vi "J1939 Workspace Tool.vi"() -> ()   [LabVIEW 2015, in "J1939 Workspace Object.lvlib"]
uses:
  J1939 Workspace Object.lvlib
  NationalInstruments.VeriStand.SystemStorage
  Shared/Types/Private Data.ctl
  Shared/Types/Error Cluster.ctl
  Shared/Types/Error Types.ctl
  Shared/J1939 Utilities/SubVIs/Convert CAN Arb ID to J1939 ID.vi
  <vilib>/NI Veristand/Execution/Workspace/NI_VS Workspace ExecutionAPI.lvlib
  Shared/J1939 Addon Shared.lvlib
  Shared/J1939 Utilities/J1939 Utilities.lvlib
  <vilib>/NI/VeriStand Addon Network Comm/Shared/NI VeriStand Addon Network Comm Shared.lvlib
panel:
  out "Device":string
  in  "Cluster":T1={"PGN"=65226, "DA"=0, "CD Path"="", "CD IP"=""}
  in  "Errors":bool
  in  "Tab Control":enum32{"DTCs", "Custom RQST", "RAW FRAME"}(tab)
  in  "Refresh Continuous":bool
  in  "Clear DTC":bool
  in  "Refresh DTCs":bool
  in  "DTCs":i32(listbox)
  in  "Addresses":string(tree)
  in  "Refresh Addresses":bool
  out "Response":string
  in  "Request":bool
  in  "PGN":u32
  in  "DA":u8(ring)
  in  "Clear Array":bool
  out "Priority":u8 format="%02x"
  out "SA":u8 format="%02x"
  out "PGN":u32 format="%06x"
  in  "Identifier":u32 format="%08x"
  in  "RAW":bool
  in  "Data":u8[](array[numeric])=[0, 0, 0, 0, 0, 0, 0, 0]
  in  "NIVS.System Definition Root":refnum<k24>
  in  "NIVS.Workspace Event":refnum<event-registration>
  in  "NIVS.Gateway IP Address":string
  # "Use this example as a template to create custom tools for the NI VeriStand Workspace. This example shows the use of the NI VeriStand API and UI controls to set and get data.\n\nRun this example by adding this VI as a Workspace Tool item. For Help adding Workspace Tool items, please reference the NI VeriStand Help."
  # "This is the file path to the VeriStand system definition file. You can read or write to the file using the System Definition API."
  # "This is the root reference to the active System Definition file. You could use this to read the configuration or populate a tree with channels. You are free to close this reference, but it will be closed for you if you don't."
  # "The SystemStorageUI .NET assembly provides controls to display data configured in the System Definition file."
  # "This is the IP Address of the VeriStand Gateway to which the Workspace is connected. Use this to open all the .NET Manager references. Usually the Gateway is running on localhost, but it could be running on a neighbor's machine."
  # "This registered string User Event is used to help instruct your tool to shut down when the Workspace is closing."
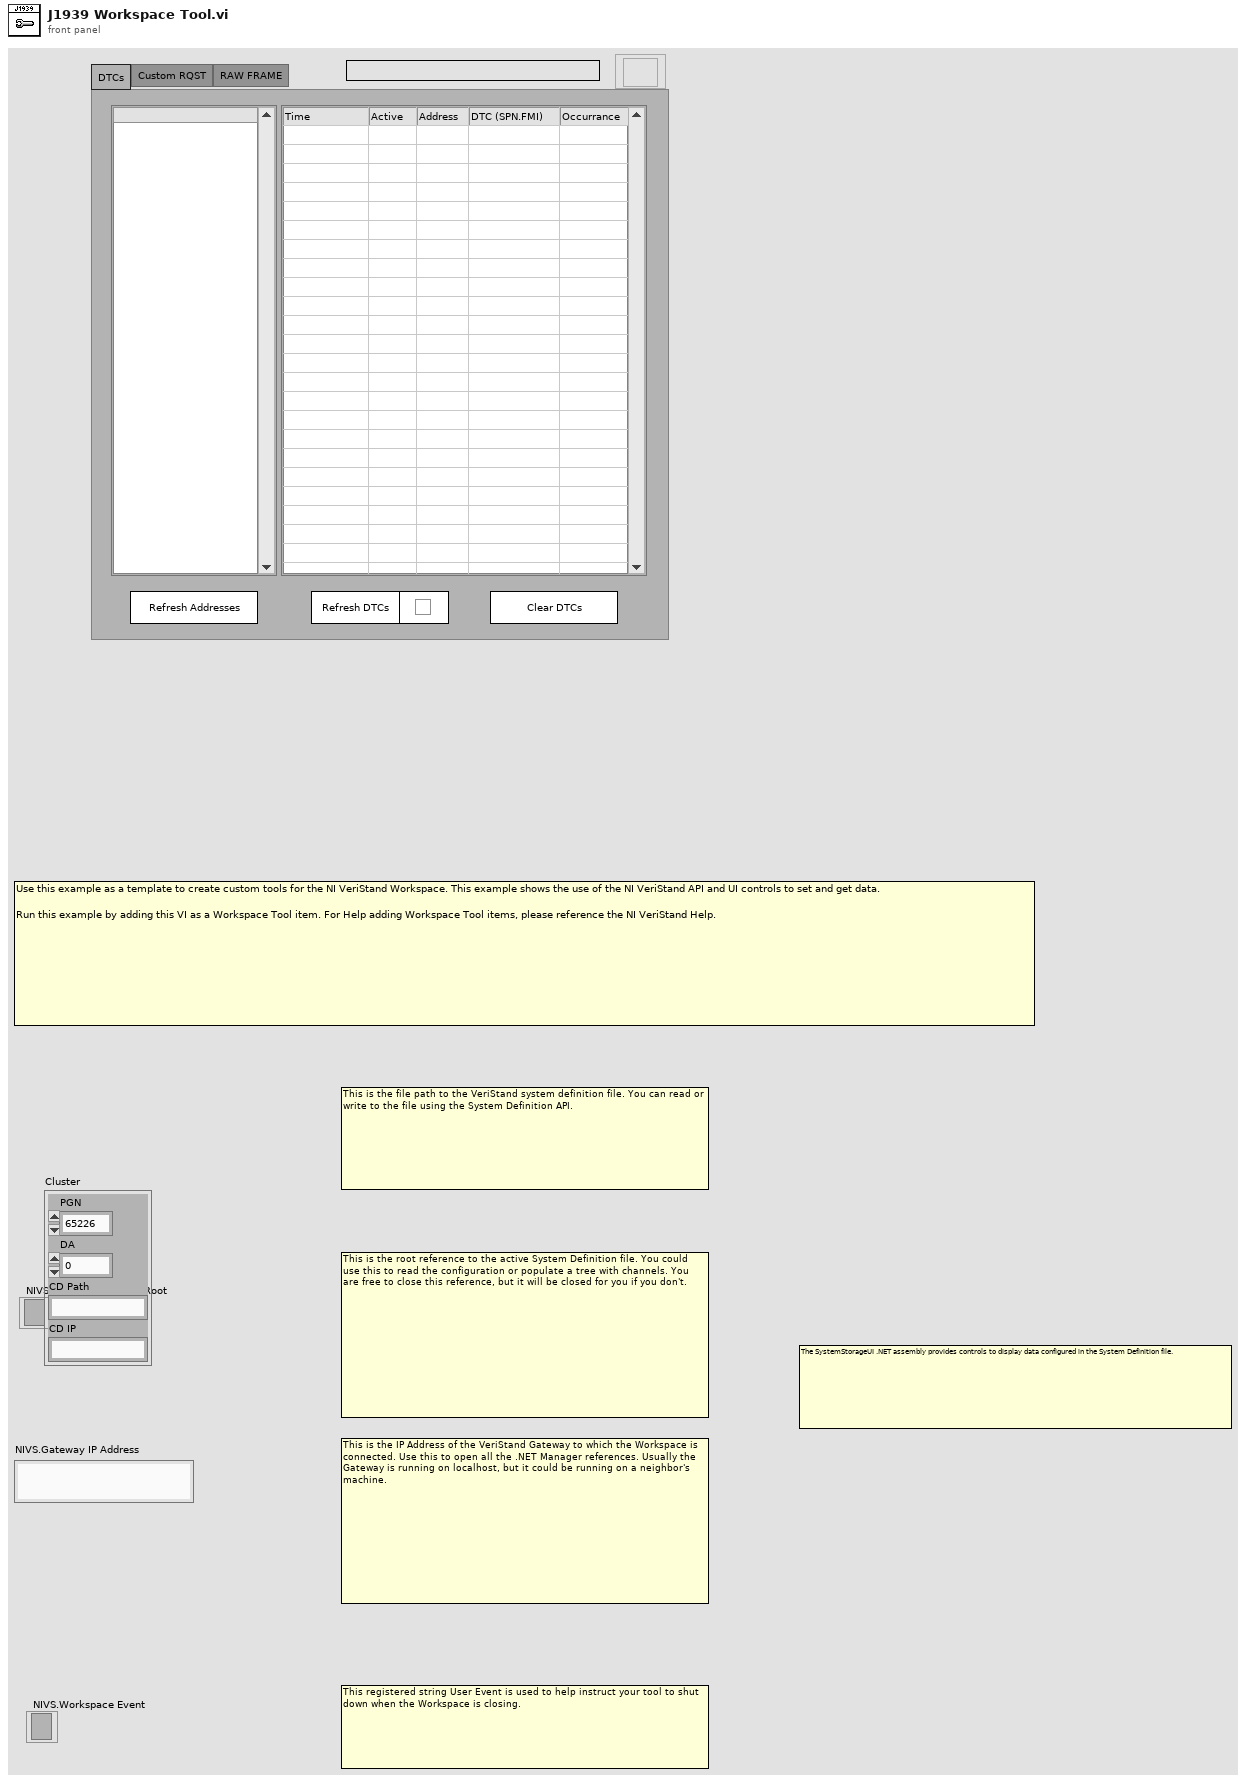
[diagram p1: front panel]
types:
  T1 = typedef "J1939 Addon Shared.lvlib/Private Data.ctl" = cluster{"PGN":u32, "DA":u8, "CD Path":string, "CD IP":string}
  T2 = typedef "J1939 Addon Shared.lvlib/Error Cluster.ctl" = cluster{"error out":errorcluster, "Enum":T3, "Address":u8, "Timestamp":timestamp}
  T3 = typedef "J1939 Addon Shared.lvlib/Error Types.ctl" = enum16{"Request", "RAW Generation", "Clear Active DTCs", "Clear Previous DTCs", "Addresses", "TLAs", "Get Active DTCs", "Get Previous DTCs"}
  T4 = typedef "NI STM.lvlib/TCP Connection Info.ctl" = cluster{"connection ID":refnum<k5>, "meta data":T5[]}
  T5 = typedef "NI STM.lvlib/MetaDataElement.ctl" = string
  T6 = typedef "NI_VS Workspace ExecutionAPI.lvlib/WorkspaceAPI.ctl" = refnum<k24>
  T7 = typedef "NI_VS Workspace ExecutionAPI.lvlib/SystemStateEventRef.ctl" = cluster{"CustDatRef":refnum<user-event>, "EvtRef":refnum<k27>, "Target State User Event":refnum<user-event>}
  T8 = typedef "NI_VS Workspace ExecutionAPI.lvlib/SystemStateRegEventRef.ctl" = refnum<event-registration>
  T9 = cluster{"NIVS.Workspace Event":refnum<event-registration>, "SystemChangeEventRef":T8}
  T10 = enum8{"Enabled", "Disabled", "Disabled and Grayed Out"}
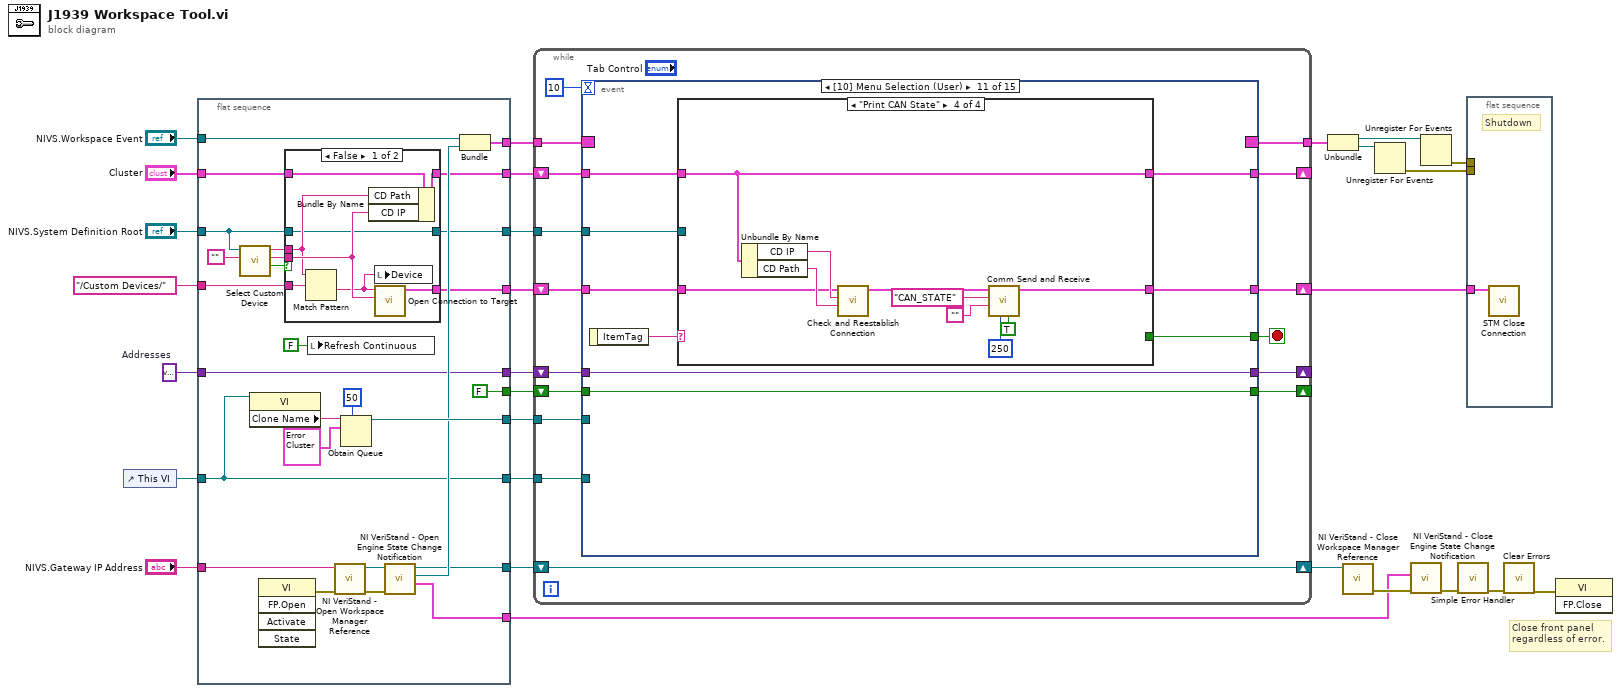
[diagram p0: block diagram]
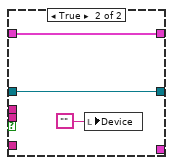
[diagram p2: hidden frame]
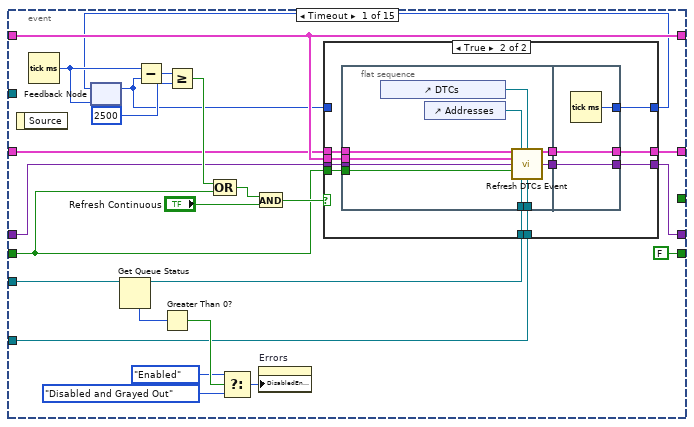
[diagram p3: hidden frame]
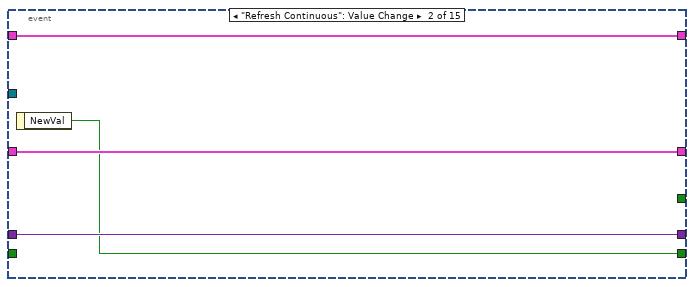
[diagram p5: hidden frame]
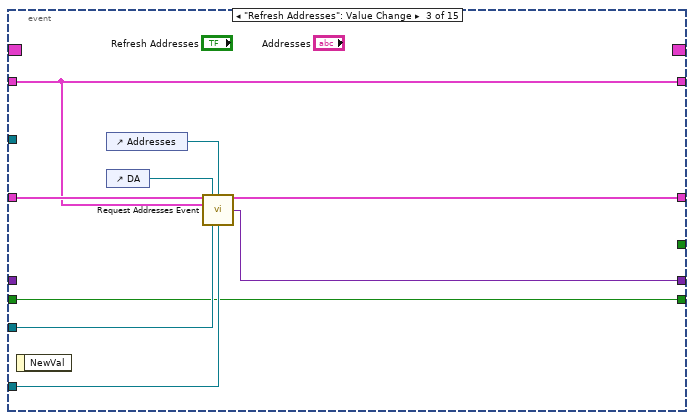
[diagram p6: hidden frame]
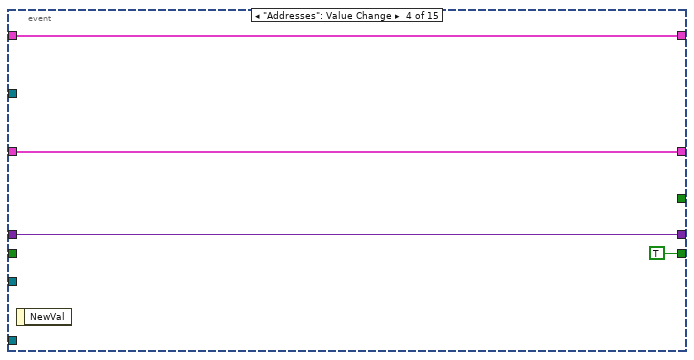
[diagram p7: hidden frame]
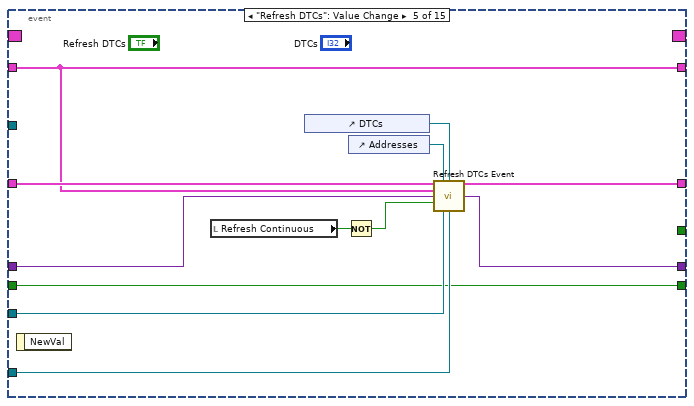
[diagram p8: hidden frame]
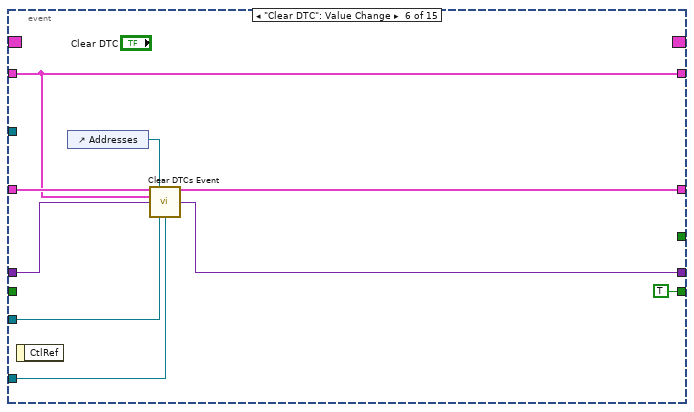
[diagram p9: hidden frame]
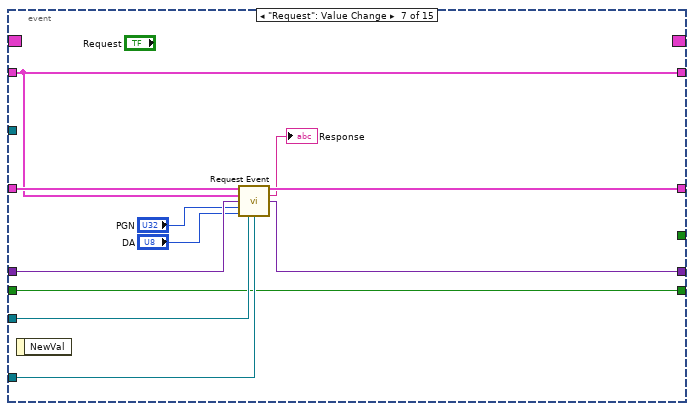
[diagram p10: hidden frame]
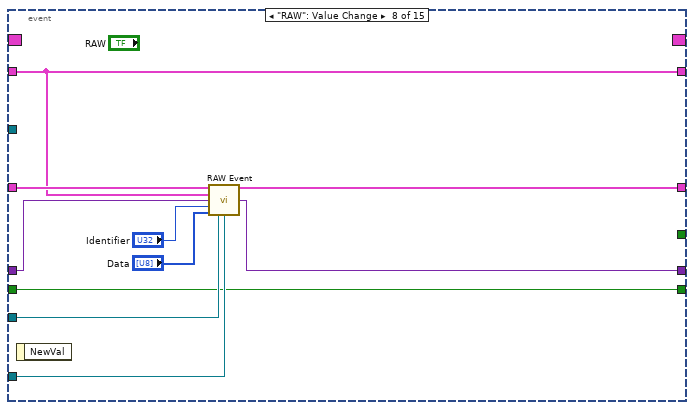
[diagram p11: hidden frame]
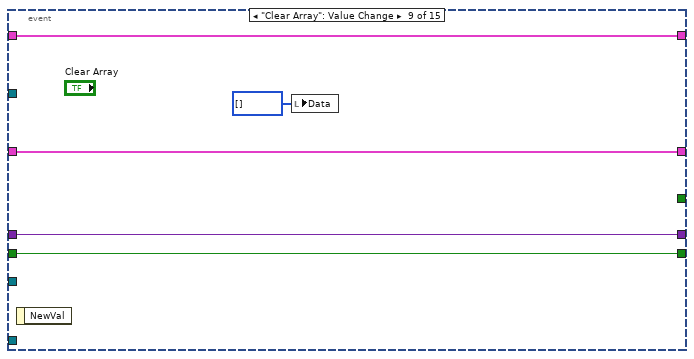
[diagram p12: hidden frame]
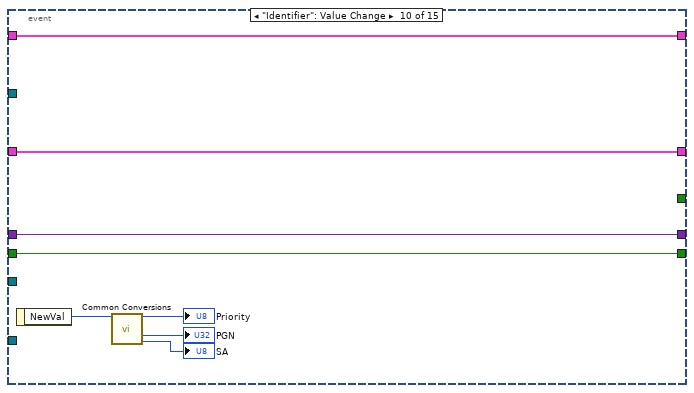
[diagram p13: hidden frame]
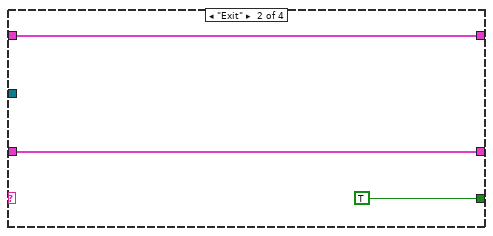
[diagram p15: hidden frame]
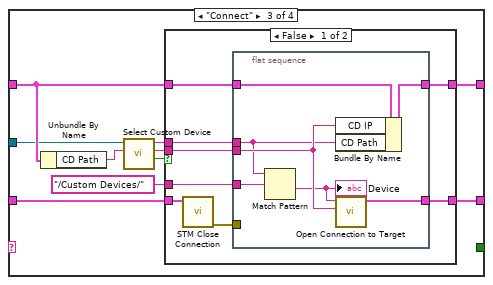
[diagram p16: hidden frame]
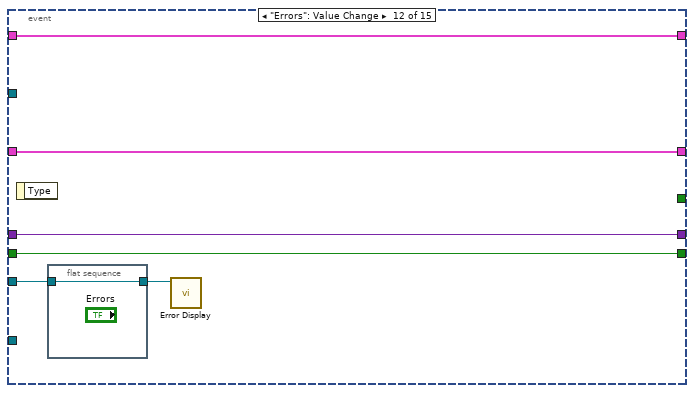
[diagram p18: hidden frame]
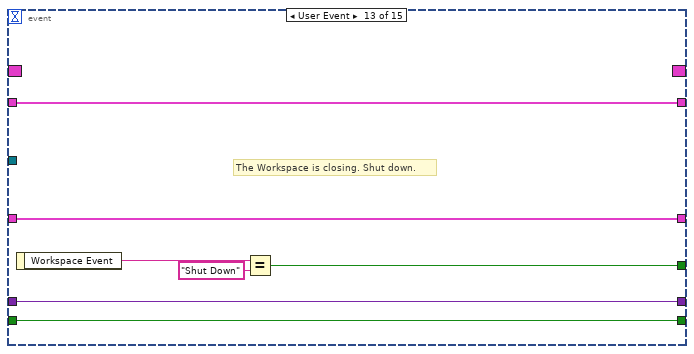
[diagram p19: hidden frame]
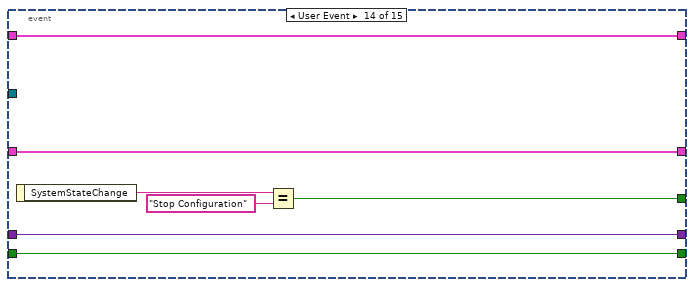
[diagram p20: hidden frame]
diagram:
  w6 = variant  # Addresses
  # "Close front panel\nregardless of error."
  n1 = control-ref of="This VI"() -> (w8:refnum<vi>)
  n2 = flat-sequence {
    tunnel: [w37] -> w28
    tunnel: [w41] -> w26
    tunnel: "NIVS.System Definition Root" -> [w31]
    tunnel: [w54] -> w25
    tunnel: [w42] -> w24
    tunnel: "NIVS.Gateway IP Address" -> [w48]
    tunnel: "NIVS.Workspace Event" -> [w46]
    tunnel: [w45] -> w20
    tunnel: [w44] -> w12
    tunnel: [w43] -> w11
    tunnel: [w39] -> w9
    tunnel: w8 -> [w42]
    tunnel: "Cluster" -> [w38]
    tunnel: w6 -> [w41]
    tunnel: [w30] -> w3
    tunnel: "/Custom Devices/" ("regular expression") -> [w35]
    tunnel: [FALSE] -> w1
    frame #0 {
      n3 = call "Select Custom Device.vi"("CD Path"="", "NIVS.System Definition Root"=w31) -> ("Cancelled?"=w32:bool, "IP Address"=w40:string, "Custom Device Path Out"=w34:string)  [unwired: 7 in]
      n4 = property class="VI"(reference=w42) -> ("Clone Name"=w55:string)  [unwired: 1 in, 2 out]
      n5 = invoke class="VI" method="FP.Open"() -> (error out=w51:errorcluster)  [unwired: 5 in, 4 out]
      n6 = case shown="False" w32 {
        tunnel: w40 -> [w63 _]
        tunnel: [w62 _] -> w39
        tunnel: w38 -> [w60 w66]
        tunnel: [w59 w66] -> w37
        tunnel: w35 -> [w58 _]
        tunnel: w34 -> [w57 _]
        tunnel: w31 -> [w56 w64]
        tunnel: [w56 w64] -> w30
        frame False {
          n7 = Match Pattern(string=w57, regular expression=w58) -> (after substring=w61:string)  [unwired: 1 in, 3 out]
          n8 = Bundle By Name(cluster=w60, "CD Path"=w57, "CD IP"=w63) -> (w59:T1)
          n9 = local write "Device"(w61) -> ()
          n10 = call "Open Connection to Target.vi"("IP Address"=w63, "TCP Service"=w61) -> ("connection info"=w62:T4)  [unwired: 8 in, 1 out]
        }
        frame True {
          n11 = local write "Device"("") -> ()
        }
      }
      n12 = local write "Refresh Continuous"(FALSE ("Refresh Continuous")) -> ()
      n13 = call <vilib>:"NI VeriStand - Open Workspace Manager Reference.vi"("error in (no error)"=w51, "Gateway IP Address (\"\": localhost)"=w48) -> ("error out"=w50:errorcluster, "WorkspaceManager"=w49:T6)  [unwired: 8 in]
      n14 = Obtain Queue(max queue size (-1, unlimited)=50, name (unnamed)=w55, element data type=T2 {"error out"={"status"=FALSE, "code"=0, "source"=""}, "Enum"=enum."Request", "Address"=0, "Timestamp"=timestamp(0 s since 1904-01-01)} ("Error Cluster")) -> (queue out=w54:refnum<queue>)  [unwired: 2 in, 2 out]
      n15 = call <vilib>:"NI VeriStand - Open Engine State Change Notification.vi"("error in (no error)"=w50, "WorkspaceManager in"=w49) -> ("SystemStateRefs"=w44:T7, "SystemChangeEventRef"=w47:T8, "WorkspaceManager out"=w43:T6)  [unwired: 6 in, 1 out]
      n16 = Bundle("NIVS.Workspace Event"=w46, "SystemChangeEventRef"=w47) -> (w45:T9)  [unwired: 1 in]
    }
  }
  n17 = while {
    tunnel: [w81] -> w17
    shift-right: [w80] -> _
    shift-left: w28 -> [w71]
    shift-right: [w78] -> w27
    shift-left: w9 -> [w79]
    shift-right: [w77] -> _
    shift-left: w26 -> [w76]
    tunnel: w25 -> [w75]
    tunnel: w24 -> [w73]
    tunnel: w20 -> [w72]
    shift-right: [w70] -> w10
    shift-left: w11 -> [w70]
    tunnel: w3 -> [w69]
    shift-right: [w68] -> _
    shift-left: w1 -> [w67]
    stop <- w82 stop-if-true
    n18 = event shown="[10] Menu Selection (User)" {
      selector: w72 -> [_ _ _ _ _ _ _ _ _ _ _ _ _ _ _]
      dyn-events: [_ _ _ _ _ _ _ _ _ _ _ _ _ _ _] -> w81
      timeout: 10 -> [_ _ _ _ _ _ _ _ _ _ _ _ _ _ _]
      tunnel: [_ _ _ _ _ _ _ _ _ _ w207 _ w268 w275 w279] -> w82
      tunnel: [w92 w137 w145 w150 w158 w166 w177 w187 w195 w205 w213 w260 w266 w272 w280] -> w80
      tunnel: w79 -> [w91 w136 w146 w149 w162 w171 w182 w192 w196 w204 w209 w262 w265 w273 w281]
      tunnel: [w90 w136 w144 w149 w159 w170 w181 w191 w196 w204 w212 w262 w265 w273 w281] -> w78
      tunnel: [w93 w135 w143 w148 w160 w168 w178 w190 w197 w203 w210 w261 w267 w274 w282] -> w77
      tunnel: w76 -> [w94 w135 _ w148 w161 w169 w179 w189 w197 w203 w210 w261 w267 w274 w282]
      tunnel: w75 -> [w106 _ w142 _ w157 w167 w180 w188 _ _ _ w258 _ _ _]
      tunnel: w73 -> [w87 _ w141 _ w156 w165 w176 w186 _ _ _ _ _ _ _]
      tunnel: w71 -> [w92 w137 w145 w150 w158 w166 w177 w187 w195 w205 w214 w260 w266 w272 w280]
      tunnel: w69 -> [_ _ _ _ _ _ _ _ _ _ w211 _ _ _ _]
      tunnel: [FALSE w134 w138 TRUE w153 TRUE w172 w183 w193 w198 w206 w257 w264 w271 w278] -> w68
      tunnel: w67 -> [w85 _ w138 _ w153 _ w172 w183 w193 w198 w206 w257 w264 w271 w278]
      event Timeout {
        n19 = event-data() -> ()  [unwired: 2 out]
        n20 = Tick Count (ms)() -> (millisecond timer value=w97:u32)
        n21 = feedback #1(w97) -> (w83:u32)
        n22 = Get Queue Status(queue=w106) -> (queue out=w88:refnum<queue>, # elements in queue=w105:i32)  [unwired: 2 in, 6 out]
        n23 = Subtract(x=w97, y=w83) -> (x-y=w95:u32)
        n24 = Greater Than 0?(x=w105) -> (x > 0?=w104:bool)
        n25 = Greater Or Equal?(x=w95, y=u32 2500) -> (x >= y?=w98:bool)
        n26 = Compound Arithmetic op=OR(w98, w85) -> (w100:bool)
        n27 = Select(t=T10."Enabled" ("Disabled"), s=w104, f=T10."Disabled and Grayed Out") -> (s? t:f=w101:T10)
        n28 = And(x=w100, y="Refresh Continuous") -> (x .and. y?=w99:bool)
        n29 = property on="Errors" class="Bool"("DisabledEnum"=w101) -> ()  [unwired: 2 in, 2 out]
        n30 = case shown="True" w99 {
          tunnel: w94 -> [w109 w120]
          tunnel: [w109 w119] -> w93
          tunnel: w91 -> [w108 w118]
          tunnel: [w108 w117] -> w90
          tunnel: w92 -> [_ w116]
          tunnel: w88 -> [_ w115]
          tunnel: w87 -> [_ w114]
          tunnel: w85 -> [_ w113]
          tunnel: [w107 w110] -> w84
          tunnel: w83 -> [w107 _]
          frame False {
          }
          frame True {
            n31 = flat-sequence {
              tunnel: w120 -> [w130]
              tunnel: w118 -> [w128]
              tunnel: w116 -> [w126]
              tunnel: w115 -> [w125]
              tunnel: w114 -> [w124]
              tunnel: w113 -> [w121]
              tunnel: [w129] -> w112
              tunnel: [w127] -> w111
              tunnel: [w132] -> w117
              tunnel: [w133] -> w119
              tunnel: w112 -> [w133]
              tunnel: w111 -> [w132]
              tunnel: [w131] -> w110
              frame #0 {
                n32 = control-ref of="DTCs"() -> (w123:refnum<vi>)
                n33 = control-ref of="Addresses"() -> (w122:refnum<vi>)
                n34 = call "Refresh DTCs Event.vi"("connection info"=w128, "Addresses"=w122, "DTCs"=w123, "State Variables"=w126, "Address Lookup Table"=w130, "To Top (T)"=w121, "Error Q"=w125, "VI Ref"=w124) -> ("connection info"=w127:T4, "Address Lookup Table Out"=w129:variant)  [unwired: 6 in]
              }
              frame #1 {
                n35 = Tick Count (ms)() -> (millisecond timer value=w131:u32)
              }
            }
          }
        }
        n36 = feedback-in #1(w84) -> ()
      }
      event "Refresh Continuous": Value Change {
        n37 = event-data() -> ("NewVal"=w134:bool)  [unwired: 1 out]
      }
      event "Refresh Addresses": Value Change {
        n38 = event-data() -> ()  [unwired: 2 out]
        n39 = control-ref of="Addresses"() -> (w139:refnum<vi>)
        n40 = control-ref of="DA"() -> (w140:refnum<vi>)
        n41 = call "Request Addresses Event.vi"("connection info"=w146, "DA"=w140, "Addresses"=w139, "State Variables"=w145, "Error Q"=w142, "VI Ref"=w141) -> ("connection info"=w144:T4, "Address Lookup Table Out"=w143:variant)  [unwired: 8 in]
      }
      event "Addresses": Value Change {
        n42 = event-data() -> ()  [unwired: 2 out]
      }
      event "Refresh DTCs": Value Change {
        n43 = event-data() -> ()  [unwired: 2 out]
        n44 = local read "Refresh Continuous"() -> (w152:bool)
        n45 = control-ref of="DTCs"() -> (w154:refnum<vi>)
        n46 = Not(x=w152) -> (.not. x?=w151:bool)
        n47 = control-ref of="Addresses"() -> (w155:refnum<vi>)
        n48 = call "Refresh DTCs Event.vi"("connection info"=w162, "Addresses"=w155, "DTCs"=w154, "State Variables"=w158, "Address Lookup Table"=w161, "To Top (T)"=w151, "Error Q"=w157, "VI Ref"=w156) -> ("connection info"=w159:T4, "Address Lookup Table Out"=w160:variant)  [unwired: 6 in]
      }
      event "Clear DTC": Value Change {
        n49 = event-data() -> ()  [unwired: 2 out]
        n50 = control-ref of="Addresses"() -> (w164:refnum<vi>)
        n51 = call "Clear DTCs Event.vi"("connection info"=w171, "Addresses"=w164, "State Variables"=w166, "Address Lookup Table"=w169, "Error Q"=w167, "VI Ref"=w165) -> ("connection info"=w170:T4, "Address Lookup Table Out"=w168:variant)  [unwired: 8 in]
      }
      event "Request": Value Change {
        n52 = event-data() -> ()  [unwired: 2 out]
        n53 = call "Request Event.vi"("connection info"=w182, "State Variables"=w177, "Address Lookup Table"=w179, "PGN"="PGN", "DA"="DA", "Error Q"=w180, "VI Ref"=w176) -> ("connection info"=w181:T4, "Response"=→"Response":string, "Address Lookup Table Out"=w178:variant)  [unwired: 6 in]
      }
      event "RAW": Value Change {
        n54 = event-data() -> ()  [unwired: 2 out]
        n55 = call "RAW Event.vi"("connection info"=w192, "State Variables"=w187, "Address Lookup Table"=w189, "Identifier"="Identifier", "Data"="Data", "Error Q"=w188, "VI Ref"=w186) -> ("connection info"=w191:T4, "Address Lookup Table Out"=w190:variant)  [unwired: 7 in]
      }
      event "Clear Array": Value Change {
        n56 = event-data() -> ()  [unwired: 2 out]
        n57 = local write "Data"(u8[] [] ("Data")) -> ()
      }
      event "Identifier": Value Change {
        n58 = event-data() -> ("NewVal"=w199:u32)  [unwired: 1 out]
        n59 = call-poly "Common Conversions.vi"("Arb ID"=w199) -> ("Priority"=→"Priority":u8, "PGN"=→"PGN":u32, "Source Address"=→"SA":u8)  [unwired: 11 in, 1 out]
      }
      event Menu Selection (User) {
        n60 = event-data() -> ("ItemTag"=w208:string)  [unwired: 1 out]
        n61 = case shown="\"Print CAN State\"" w208 {
          tunnel: w214 -> [w216 w219 w224 w248]
          tunnel: [w216 w219 w220 w248] -> w213
          tunnel: [w215 w218 w221 w249] -> w212
          tunnel: w211 -> [_ _ w223 _]
          tunnel: w209 -> [w215 w218 w222 w250]
          tunnel: [_ TRUE _ _] -> w207
          frame Default {
          }
          frame "Exit" {
          }
          frame "Connect" {
            n62 = Unbundle By Name(w224) -> ("CD Path"=w228:string)
            n63 = call "Select Custom Device.vi"("CD Path"=w228, "NIVS.System Definition Root"=w223) -> ("Cancelled?"=w225:bool, "IP Address"=w229:string, "Custom Device Path Out"=w226:string)  [unwired: 7 in]
            n64 = case shown="False" w225 {
              tunnel: w224 -> [w237 w246]
              tunnel: [w236 w245] -> w221
              tunnel: [w235 w246] -> w220
              tunnel: w229 -> [w234 _]
              tunnel: "/Custom Devices/" ("regular expression") -> [w233 _]
              tunnel: w226 -> [w232 _]
              tunnel: w222 -> [w231 w245]
              frame False {
                n65 = call "STM Close Connection.vi"("connection info"=w231) -> ("error out"=w230:errorcluster)  [unwired: 10 in]
                n66 = flat-sequence {
                  tunnel: w237 -> [w244]
                  tunnel: [w243] -> w236
                  tunnel: [w242] -> w235
                  tunnel: w234 -> [w241]
                  tunnel: w233 -> [w240]
                  tunnel: w232 -> [w239]
                  tunnel: w230 -> [_]
                  frame #0 {
                    n67 = Match Pattern(string=w239, regular expression=w240) -> (after substring=w238:string)  [unwired: 1 in, 3 out]
                    "Device" <- w238
                    n68 = Bundle By Name(cluster=w244, "CD IP"=w241, "CD Path"=w239) -> (w242:T1)
                    n69 = call "Open Connection to Target.vi"("IP Address"=w241, "TCP Service"=w238) -> ("connection info"=w243:T4)  [unwired: 8 in, 1 out]
                  }
                }
              }
              frame True {
              }
            }
          }
          frame "Print CAN State" {
            n70 = Unbundle By Name(w248) -> ("CD IP"=w255:string, "CD Path"=w254:string)
            n71 = call "Check and Reestablish Connection.vi"("CD Path"=w254, "IP Address"=w255, "connection info"=w250) -> ("connection info"=w253:T4)  [unwired: 7 in, 1 out]
            n72 = call <vilib>:"Comm Send and Receive.vi"("Resp Required?"=TRUE, "Timeout (ms)"=u32 250 ("Timeout ms (5000)"), "Data"="", "Name"="CAN_STATE", "connection info"=w253) -> ("connection info"=w249:T4)  [unwired: 3 in, 3 out]
          }
        }
      }
      event "Errors": Value Change {
        n73 = event-data() -> ()  [unwired: 2 out]
        n74 = flat-sequence {
          tunnel: [w263] -> w259
          tunnel: w258 -> [w263]
          frame #0 {
          }
        }
        n75 = call "Error Display.vi"("queue out"=w259) -> ()  [unwired: 11 in]
      }
      event User Event {
        # "The Workspace is closing. Shut down."
        n76 = event-data() -> ("Workspace Event"=w269:string)  [unwired: 1 out]
        n77 = Equal?(x=w269, y="Shut Down") -> (x = y?=w268:bool)
      }
      event User Event {
        n78 = event-data() -> ("SystemStateChange"=w276:string)  [unwired: 1 out]
        n79 = Equal?(x=w276, y="Stop Configuration") -> (x = y?=w275:bool)
      }
      event Panel Close? {
        w279 = TRUE ("Discard?")
        n80 = event-data() -> ()  [unwired: 2 out]
        n81 = event-data("Discard?"=w279) -> ()  [unwired: 1 in, 1 out]
      }
    }
  }
  n82 = Unbundle(w17) -> ("NIVS.Workspace Event"=w19:refnum<event-registration>, "SystemChangeEventRef"=w18:T8)
  n83 = call <vilib>:"NI VeriStand - Close Workspace Manager Reference.vi"("WorkspaceManager"=w10) -> ("error out"=w13:errorcluster)  [unwired: 10 in]
  n84 = Unregister For Events(event registration refnum=w18) -> (error out=w4:errorcluster)  [unwired: 1 in]
  n85 = call <vilib>:"NI VeriStand - Close Engine State Change Notification.vi"("error in (no error)"=w13, "SystemStateRefs"=w12) -> ("error out"=w14:errorcluster)  [unwired: 9 in]
  n86 = Unregister For Events(event registration refnum=w19) -> (error out=w5:errorcluster)  [unwired: 1 in]
  n87 = call <vilib>:"Simple Error Handler.vi"("error in (no error)"=w14) -> ("error out"=w15:errorcluster)  [unwired: 4 in, 4 out]
  n88 = flat-sequence {
    tunnel: w27 -> [w283]
    tunnel: w5 -> [_]
    tunnel: w4 -> [_]
    frame #0 {
      # "Shutdown"
      n89 = call "STM Close Connection.vi"("connection info"=w283) -> ()  [unwired: 10 in, 1 out]
    }
  }
  n90 = call <vilib>:"Clear Errors.vi"("error in (no error)"=w15) -> ("error out"=w16:errorcluster)  [unwired: 5 in, 1 out]
  n91 = invoke class="VI" method="FP.Close"(error in=w16) -> ()  [unwired: 2 in, 3 out]
